vi "NetCDFLabviewDemo.vi"(5 "NetCDF File:":path) -> ()   [LabVIEW 2016]
uses:
  DemoSubVIs/XControls/ArrayTree/ArrayTree.xctl
  DemoSubVIs/XControls/PairTable/PairTable.xctl
panel:
  out "var-lowst-dim name pair":cluster{"name":string, "name":string}[](array[cluster])
  out "DataArr":dbl[][](array[numeric])
  out "Var's Attritutes:":string="No attibutes" caption="valtime's attributes:"
  in  "选项卡控件":enum32{"Global ", "Detail"}(tab)
  out "Global Attritutes":cluster{"c":string, "l":string}[](xcontrol)
  out "Attritutes":cluster{"c":string, "l":string}[](xcontrol)
  out "Variable":T1(xcontrol)
  out "XY图":cluster{dbl[], "value":dbl[]}[](graph) caption="H[0] 's graph"
  in  "ViewPic":bool
  out "Text Variable":string caption="datetime[0](dump text)"
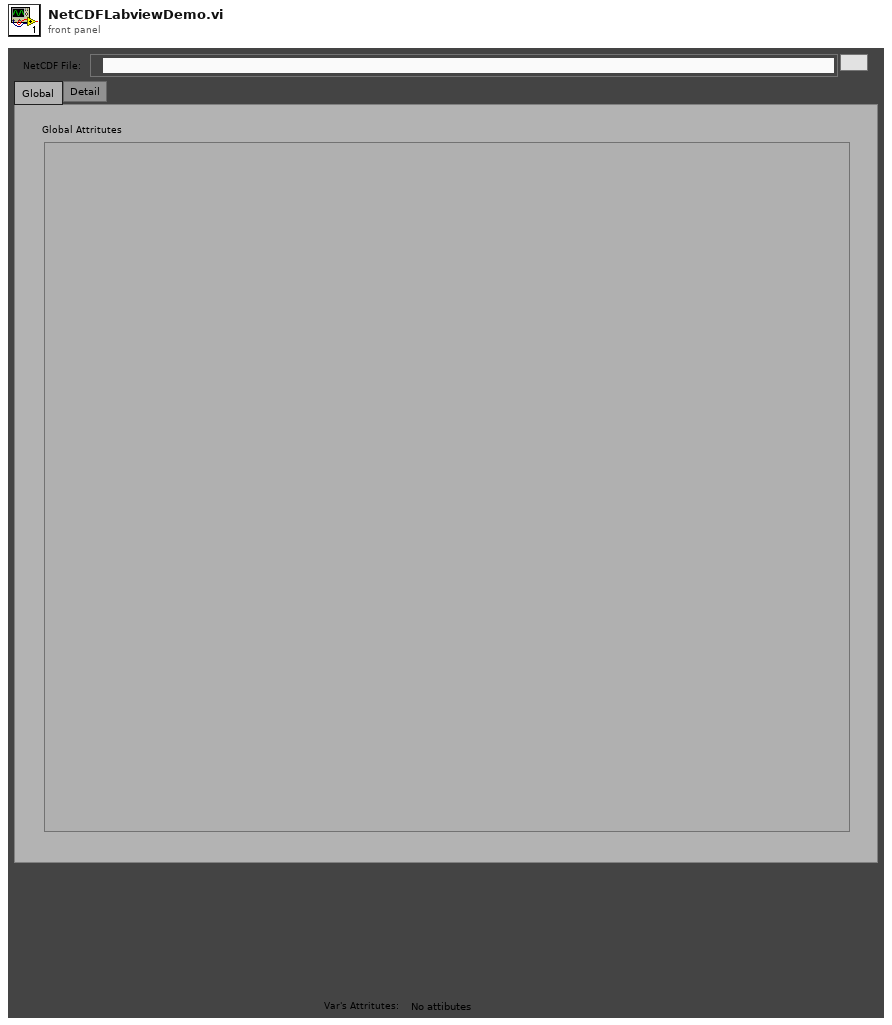
[diagram p1: front panel]
types:
  T1 = cluster{"TopLevelItemName":string, "ChildItemArr":cluster{"ChildDimName":string, "ChildDimSize":u64}[]}[]
  T2 = cluster{"TopLevelItemName":string, "ChildItemArr":cluster{"ChildDimName":string, "ChildDimSize":u64}[]}
  T3 = cluster{"xsz":u64, "shape":u64[], "dsizes":u64[], "name":string, "dimids":u64[], "NC_attrarray":cluster{"xsz":u64, "name":string, "nc_type":u16, "nelems":u64, "xvalue":string}[], "nc_type":enum16{"NC_NAT", "NC_BYTE", "NC_CHAR", "NC_SHORT", "NC_INT", "NC_FLOAT", "NC_DOUBLE"}, "len":u64, "begin":u64}
  T4 = cluster{"xsz":u64, "shape":u64[], "dsizes":u64[], "name":string, "dimids":u64[], "NC_attrarray":cluster{"xsz":u64, "name":string, "nc_type":u16, "nelems":u64, "xvalue":string}[], "nc_type":enum16{"NC_NAT", "NC_BYTE", "NC_CHAR", "NC_SHORT", "NC_INT", "NC_FLOAT", "NC_DOUBLE"}, "len":u64, "begin":u64}[]
  T5 = cluster{"xsz":u64, "name":string, "nc_type":u16, "nelems":u64, "xvalue":string}[]
  T6 = cluster{"numrecs":u64, "dims":cluster{"name":string, "size":u64}[], "attrs":cluster{"xsz":u64, "name":string, "nc_type":u16, "nelems":u64, "xvalue":string}[], "vars":cluster{"xsz":u64, "shape":u64[], "dsizes":u64[], "name":string, "dimids":u64[], "NC_attrarray":cluster{"xsz":u64, "name":string, "nc_type":u16, "nelems":u64, "xvalue":string}[], "nc_type":enum16{"NC_NAT", "NC_BYTE", "NC_CHAR", "NC_SHORT", "NC_INT", "NC_FLOAT", "NC_DOUBLE"}, "len":u64, "begin":u64}[]}
  T7 = enum16{"NC_NAT", "NC_BYTE", "NC_CHAR", "NC_SHORT", "NC_INT", "NC_FLOAT", "NC_DOUBLE"}
  T8 = cluster{"name":string, cluster{"name":string, "数值":u64}[]}[]
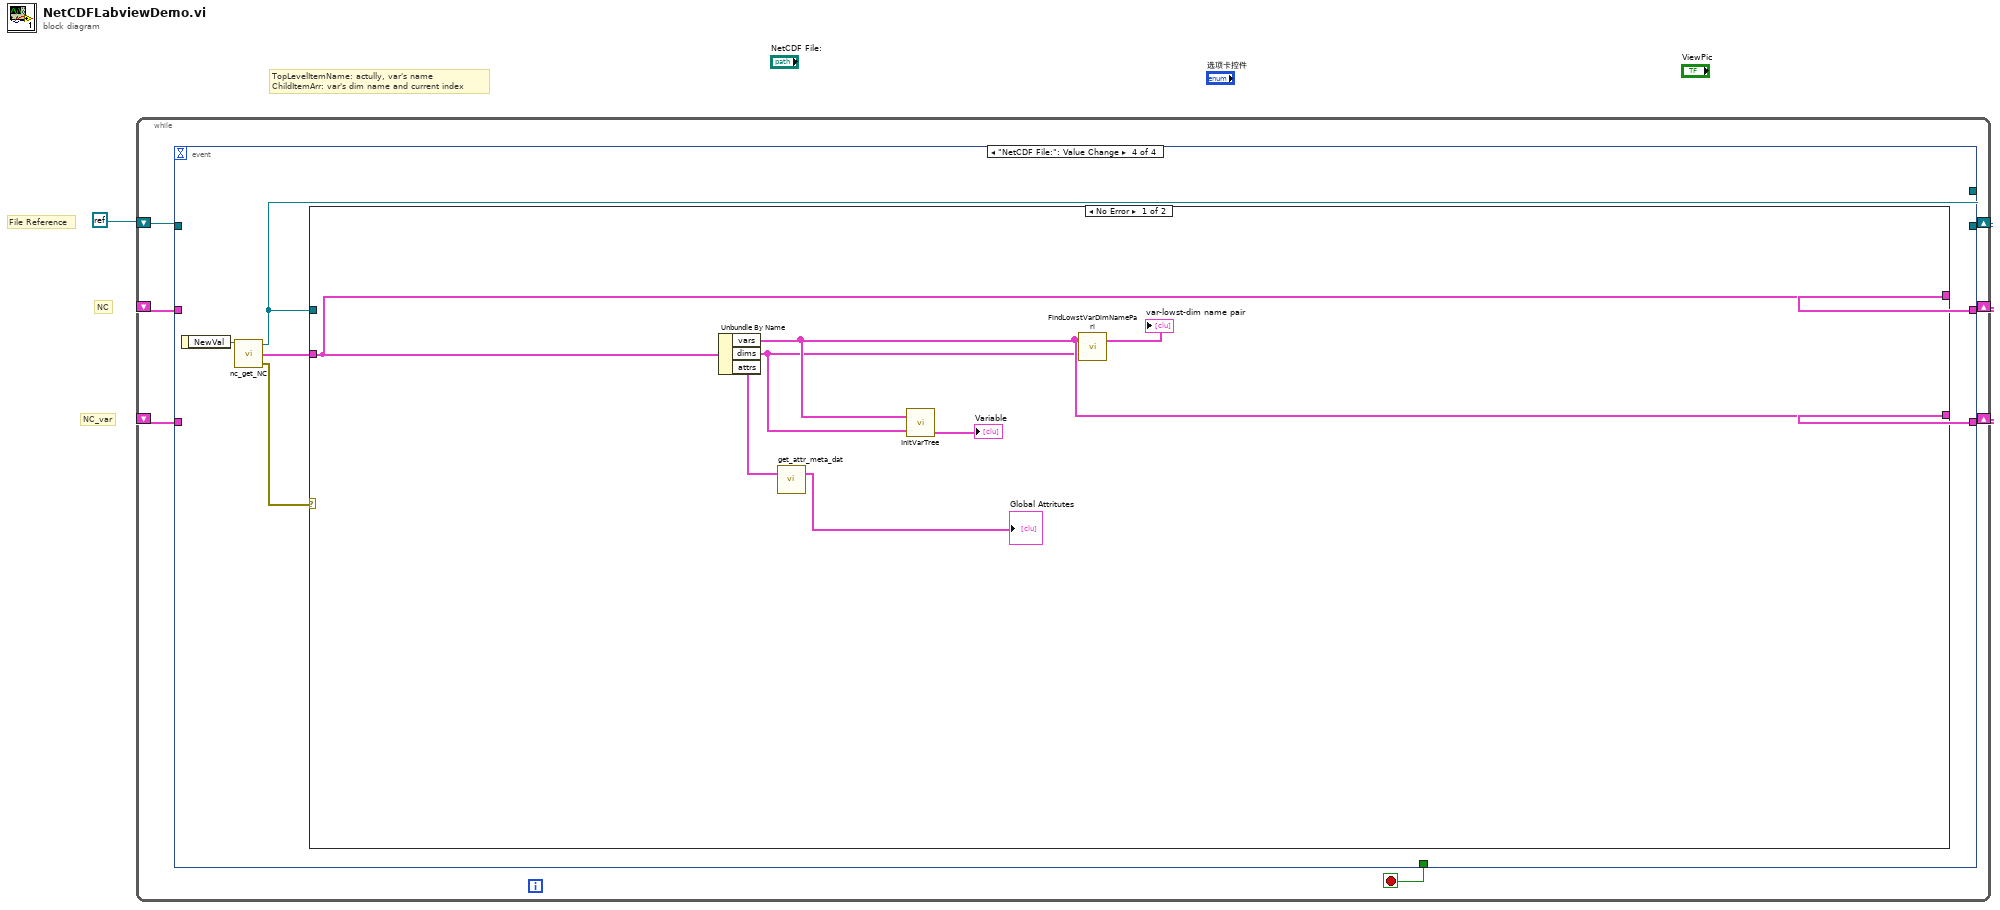
[diagram p0: block diagram]
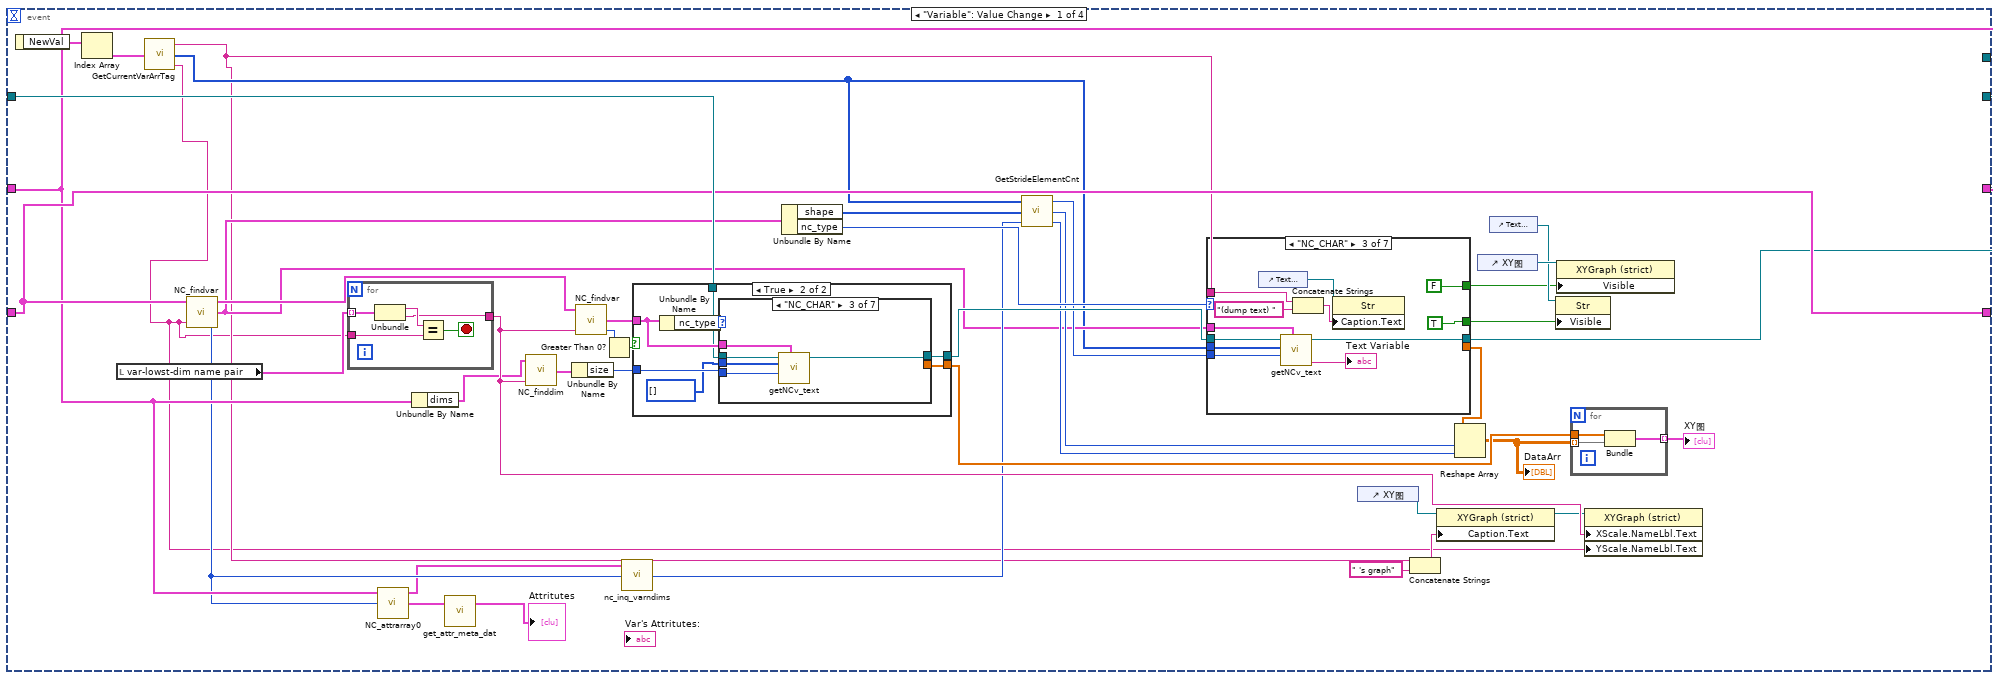
[diagram p2: hidden frame]
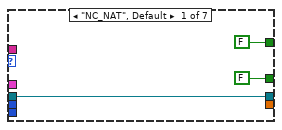
[diagram p3: hidden frame]
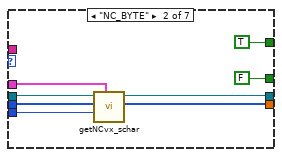
[diagram p4: hidden frame]
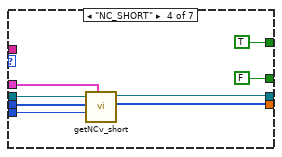
[diagram p5: hidden frame]
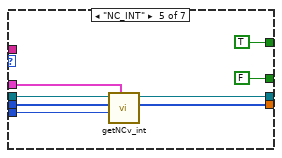
[diagram p6: hidden frame]
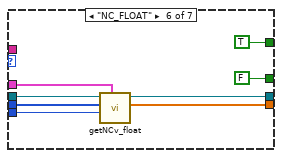
[diagram p7: hidden frame]
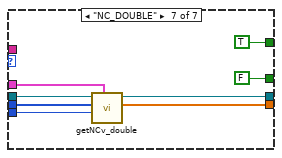
[diagram p8: hidden frame]
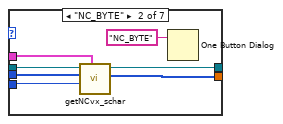
[diagram p11: hidden frame]
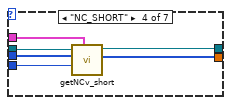
[diagram p12: hidden frame]
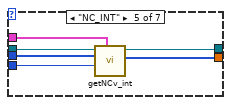
[diagram p13: hidden frame]
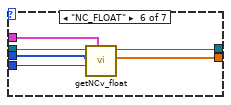
[diagram p14: hidden frame]
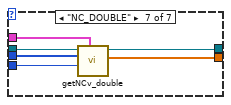
[diagram p15: hidden frame]
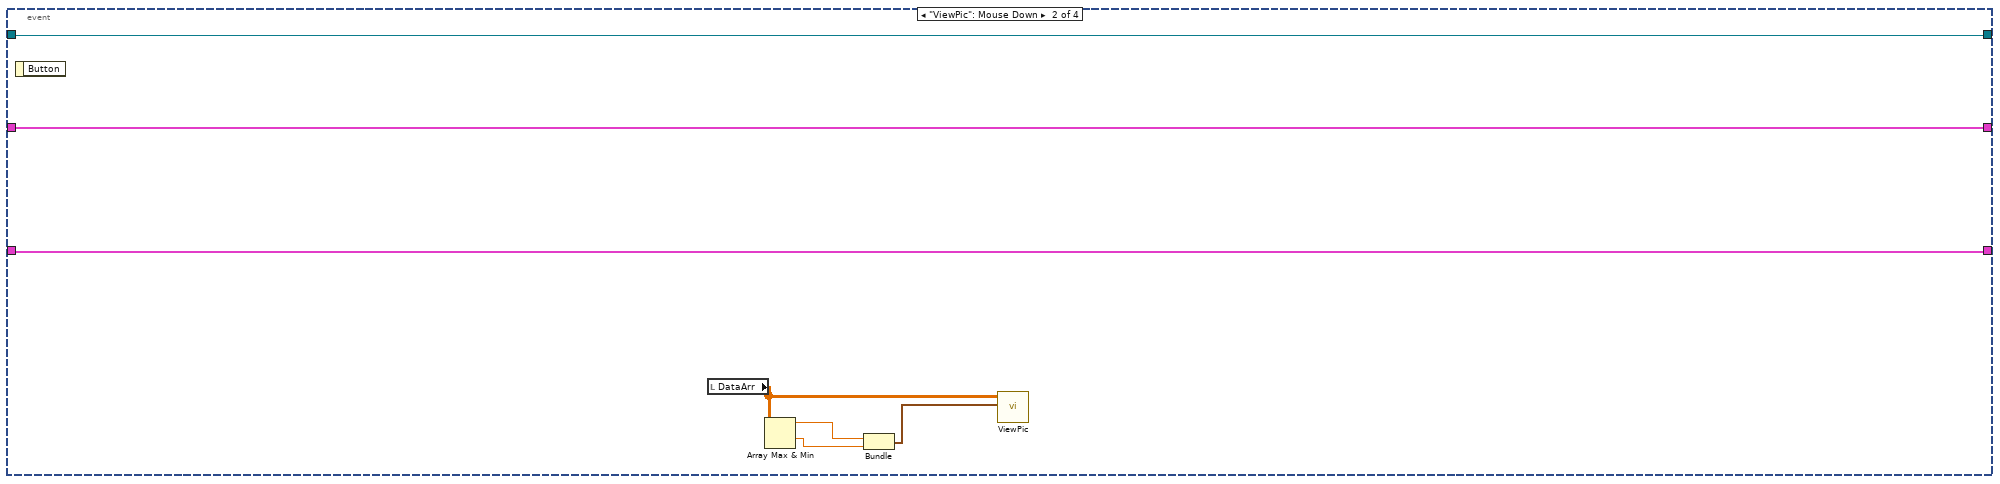
[diagram p16: hidden frame]
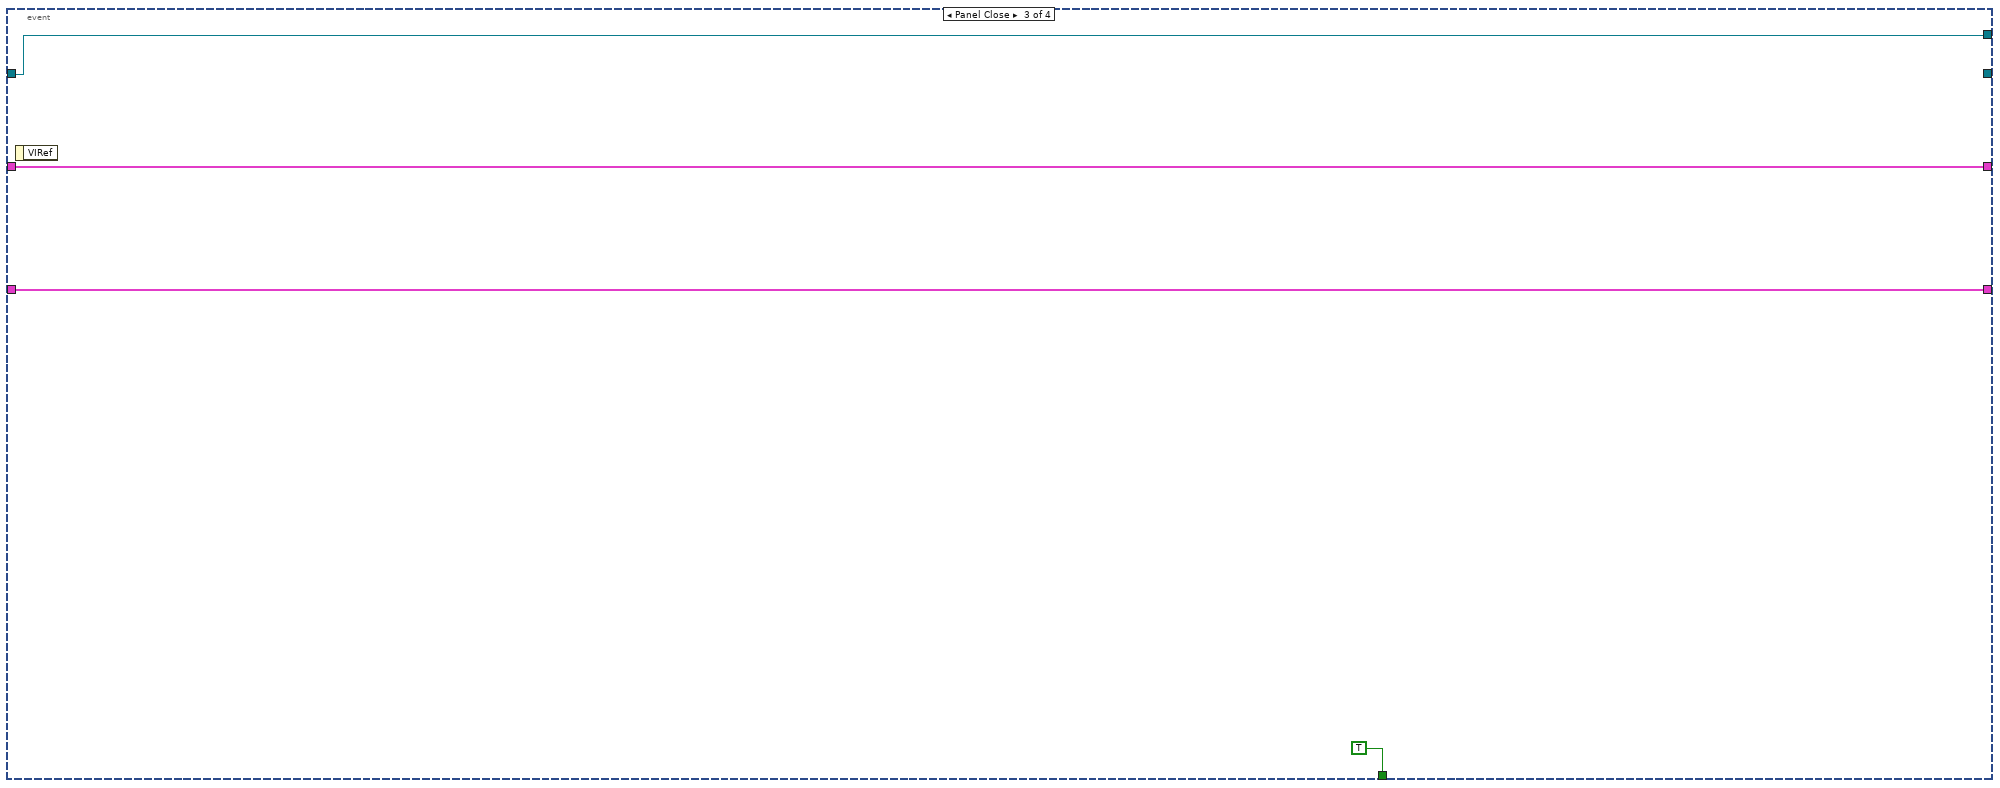
[diagram p17: hidden frame]
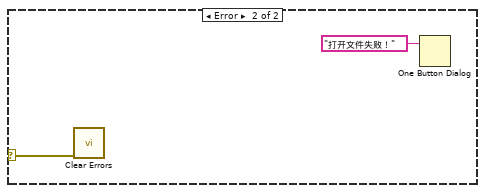
[diagram p18: hidden frame]
diagram:
  # "TopLevelItemName: actully, var's name\nChildItemArr: var's dim name and current index"
  # "File Reference"
  # "NC_var"
  # "NC"
  n1 = while {
    shift-right: [w3] -> _
    shift-left: refnum<k0> refnum -> [w6]
    shift-right: [w5] -> _
    shift-left: _ -> [w7]
    shift-right: [w4] -> _
    shift-left: _ -> [w8]
    stop <- w2 stop-if-true
    n2 = event shown="[3] \"NetCDF File:\": Value Change" {
      selector: _ -> [_ _ _ _]
      dyn-events: _ -> [_ _ _ _]
      timeout: _ -> [_ _ _ _]
      tunnel: w6 -> [w49 w162 w171 _]
      tunnel: w8 -> [w48 w164 w169 _]
      tunnel: w7 -> [w47 w163 w170 _]
      tunnel: [w47 w163 w170 w174] -> w5
      tunnel: [w48 w164 w169 w177] -> w4
      tunnel: [w46 w162 _ w173] -> w3
      tunnel: [_ _ TRUE _] -> w2
      tunnel: [_ _ w171 _] -> _
      event "Variable": Value Change {
        n3 = event-data() -> ("NewVal"=w50:T1)  [unwired: 1 out]
        n4 = Index Array(array=w50) -> (element=w44:T2)  [unwired: 1 in]
        n5 = local read "var-lowst-dim name pair"() -> (w12:cluster{"name":string, "name":string}[])
        n6 = call "GetCurrentVarArrTag.vi"("VarIndexArr"=w44) -> ("CurrentArrayTag"=w11:string, "IndexTagArr"=w14:u64[], "TopLevelItemName"=w10:string)
        n7 = call "NC_findvar.vi"("name"=w10, "NC_vararray"=w48) -> ("varid"=w34:i32, "NC_var"=w15:T3, "NC_vararray  out"=w43:T4)  [unwired: 1 out]
        n8 = for {
          tunnel: w12 -> [w159] mode=indexing
          tunnel: w10 -> [w161]
          tunnel: [w157] -> w41
          stop <- w160 stop-if-true
          n9 = Unbundle(w159) -> ("name"=w158:string, "name"=w157:string)
          n10 = Equal?(x=w158, y=w161) -> (x = y?=w160:bool)
        }
        n11 = call "NC_attrarray0.vi"("varid"=w34, "NC"=w47) -> ("NC_attrarray"=w36:T5, "NC Out"=w32:T6)  [unwired: 1 in, 1 out]
        n12 = Unbundle By Name(w47) -> ("dims"=w35:cluster{"name":string, "size":u64}[])
        n13 = call "get_attr_meta_dat.vi"("NC_attrarray"=w36) -> ("NC_attr_meta_data_arr"=→"Attritutes":cluster{"name":string, "xvalue":string}[])  [unwired: 2 out]
        n14 = call "NC_finddim.vi"("name"=w41, "NC_dimarray"=w35) -> ("NC_dim"=w42:cluster{"name":string, "size":u64})  [unwired: 3 out]
        n15 = Unbundle By Name(w42) -> ("size"=w40:u64)
        n16 = call "NC_findvar.vi"("name"=w41, "NC_vararray"=w43) -> ("varid"=w31:i32, "NC_var"=w39:T3)  [unwired: 2 out]
        n17 = Greater Than 0?(x=w31) -> (x > 0?=w30:bool)
        n18 = call "nc_inq_varndims.vi"("varid"=w34, "NC"=w32) -> ("ndims"=w33:i32)  [unwired: 1 in, 2 out]
        n19 = case shown="True" w30 {
          tunnel: w40 -> [w110 w118]
          tunnel: w39 -> [_ w117]
          tunnel: [w109 w116] -> w38
          tunnel: [w111 w115] -> w37
          tunnel: w49 -> [w111 w114]
          frame False {
            n20 = for {
              N: w110 -> [_]
              tunnel: [w112] -> w109 mode=indexing
              i -> [w112]
            }
          }
          frame True {
            n21 = Unbundle By Name(w117) -> ("nc_type"=w119:T7)
            n22 = case shown="\"NC_CHAR\"" w119 {
              tunnel: [_ w124 _ w137 w142 w147 w153] -> w116
              tunnel: w114 -> [w120 w126 w131 w138 w144 w150 w156]
              tunnel: w118 -> [_ w122 w130 w136 w143 w149 w155]
              tunnel: w117 -> [_ w125 w132 w135 w141 w148 w154]
              tunnel: [w120 w123 w129 w134 w140 w146 w152] -> w115
              tunnel: u64[] [] ("start") -> [_ w121 w128 w133 w139 w145 w151]
              frame "NC_NAT", Default {
              }
              frame "NC_BYTE" {
                n23 = call "getNCvx_schar.vi"("NC_var"=w125, "nelems"=w122, "start"=w121, "refnum"=w126) -> ("value"=w124:i8[], "refnum out"=w123:refnum<file>)  [unwired: 1 in, 2 out]
                n24 = One Button Dialog(message="NC_BYTE" ("消息")) -> ()  [unwired: 2 out]
              }
              frame "NC_CHAR" {
                n25 = call "getNCv_text.vi"("NC_var"=w132, "nelems"=w130, "start"=w128, "refnum"=w131) -> ("refnum out"=w129:refnum<file>)  [unwired: 1 in, 3 out]
              }
              frame "NC_SHORT" {
                n26 = call "getNCv_short.vi"("NC_var"=w135, "nelems"=w136, "start"=w133, "refnum"=w138) -> ("value"=w137:i16[], "refnum out"=w134:refnum<file>)  [unwired: 1 in, 2 out]
              }
              frame "NC_INT" {
                n27 = call "getNCv_int.vi"("NC_var"=w141, "nelems"=w143, "start"=w139, "refnum"=w144) -> ("value"=w142:i32[], "refnum out"=w140:refnum<file>)  [unwired: 1 in, 2 out]
              }
              frame "NC_FLOAT" {
                n28 = call "getNCv_float.vi"("NC_var"=w148, "nelems"=w149, "start"=w145, "refnum"=w150) -> ("value"=w147:sgl[], "refnum out"=w146:refnum<file>)  [unwired: 1 in, 2 out]
              }
              frame "NC_DOUBLE" {
                n29 = call "getNCv_double.vi"("NC_var"=w154, "nelems"=w155, "start"=w151, "refnum"=w156) -> ("value"=w153:dbl[], "refnum out"=w152:refnum<file>)  [unwired: 1 in, 2 out]
              }
            }
          }
        }
        n30 = Unbundle By Name(w15) -> ("shape"=w13:u64[], "nc_type"=w45:T7)
        n31 = call "GetStrideElementCnt.vi"("ndims"=w33, "shape"=w13, "CurrentIndex"=w14) -> ("shape[i-1]"=w29:u64, "shape[i-2]"=w28:u64, "strideElementCnt"=w16:u64)
        n32 = case shown="\"NC_CHAR\"" w45 {
          tunnel: [_ w60 _ w83 w89 w96 w104] -> w27
          tunnel: w37 -> [w56 w64 w74 w84 w92 w100 w108]
          tunnel: w16 -> [_ w61 w72 w82 w90 w98 w106]
          tunnel: w11 -> [_ _ w68 _ _ _ _]
          tunnel: w14 -> [_ w62 w73 w80 w91 w99 w107]
          tunnel: w15 -> [_ w63 w75 w81 w88 w97 w105]
          tunnel: [w56 w59 w70 w79 w87 w95 w103] -> w46
          tunnel: [FALSE ("可见") TRUE ("可见") FALSE ("可见") TRUE ("可见") TRUE ("可见") TRUE ("可见") TRUE ("可见")] -> w20
          tunnel: [FALSE ("可见") FALSE ("可见") TRUE ("可见") FALSE ("可见") FALSE ("可见") FALSE ("可见") FALSE ("可见")] -> w19
          frame "NC_NAT", Default {
          }
          frame "NC_BYTE" {
            n33 = call "getNCvx_schar.vi"("NC_var"=w63, "nelems"=w61, "start"=w62, "refnum"=w64) -> ("value"=w60:i8[], "refnum out"=w59:refnum<file>)  [unwired: 1 in, 2 out]
          }
          frame "NC_CHAR" {
            n34 = control-ref of="Text Variable"() -> (w76:refnum<vi>)
            n35 = call "getNCv_text.vi"("NC_var"=w75, "nelems"=w72, "start"=w73, "refnum"=w74) -> ("value"=→"Text Variable":string, "refnum out"=w70:refnum<file>)  [unwired: 1 in, 2 out]
            n36 = Concatenate Strings(w68, "(dump text) " ("字符串")) -> (w67:string)
            n37 = property class="Str"(reference=w76, "Caption.Text"=w67) -> ()  [unwired: 1 in, 2 out]
          }
          frame "NC_SHORT" {
            n38 = call "getNCv_short.vi"("NC_var"=w81, "nelems"=w82, "start"=w80, "refnum"=w84) -> ("value"=w83:i16[], "refnum out"=w79:refnum<file>)  [unwired: 1 in, 2 out]
          }
          frame "NC_INT" {
            n39 = call "getNCv_int.vi"("NC_var"=w88, "nelems"=w90, "start"=w91, "refnum"=w92) -> ("value"=w89:i32[], "refnum out"=w87:refnum<file>)  [unwired: 1 in, 2 out]
          }
          frame "NC_FLOAT" {
            n40 = call "getNCv_float.vi"("NC_var"=w97, "nelems"=w98, "start"=w99, "refnum"=w100) -> ("value"=w96:sgl[], "refnum out"=w95:refnum<file>)  [unwired: 1 in, 2 out]
          }
          frame "NC_DOUBLE" {
            n41 = call "getNCv_double.vi"("NC_var"=w105, "nelems"=w106, "start"=w107, "refnum"=w108) -> ("value"=w104:dbl[], "refnum out"=w103:refnum<file>)  [unwired: 1 in, 2 out]
          }
        }
        n42 = control-ref of="XY图"() -> (w26:refnum<vi>)
        n43 = Concatenate Strings(w11, " 's graph" ("字符串")) -> (w17:string)
        n44 = property class="XYGraph (strict)"(reference=w26, "Caption.Text"=w17) -> (reference out=w23:refnum<vi>)  [unwired: 1 in, 1 out]
        n45 = Reshape Array(w27, w28, w29) -> (w25:dbl[][])
        "DataArr" <- w25
        n46 = control-ref of="XY图"() -> (w22:refnum<vi>)
        n47 = control-ref of="Text Variable"() -> (w21:refnum<vi>)
        n48 = property class="Str"(reference=w21, "Visible"=w19) -> ()  [unwired: 1 in, 2 out]
        n49 = property class="XYGraph (strict)"(reference=w22, "Visible"=w20) -> ()  [unwired: 1 in, 2 out]
        n50 = for {
          tunnel: w25 -> [w52] mode=indexing
          tunnel: [w53] -> w24 mode=indexing
          tunnel: w38 -> [w51]
          n51 = Bundle("value"=w51, "value"=w52) -> (w53:cluster{"value":dbl[], "value":dbl[]})  [unwired: 1 out]
        }
        "XY图" <- w24
        n52 = property class="XYGraph (strict)"(reference=w23, "XScale.NameLbl.Text"=w41, "YScale.NameLbl.Text"=w10) -> ()  [unwired: 1 in, 2 out]
      }
      event "ViewPic": Mouse Down {
        n53 = event-data() -> ()  [unwired: 2 out]
        n54 = local read "DataArr"() -> (w168:dbl[][])
        n55 = Array Max & Min(array=w168) -> (max value=w167:dbl, min value=w166:dbl)  [unwired: 2 out]
        n56 = Bundle(w167, w166) -> (w165:cluster{dbl, dbl})  [unwired: 1 out]
        n57 = call "ViewPic.vi"("VarRange"=w165, "Data"=w168) -> ()  [unwired: 1 in, 9 out]
      }
      event Panel Close {
        n58 = event-data() -> ()  [unwired: 2 out]
      }
      event "NetCDF File:": Value Change {
        n59 = event-data() -> ("NewVal"=w178:path)  [unwired: 1 out]
        n60 = call "nc_get_NC.vi"("FilePath"=w178) -> ("ErrorOut"=w176:errorcluster, "NC"=w175:T6, "refnum out"=w173:refnum<file>)  [unwired: 1 in, 1 out]
        n61 = case shown="No Error" w176 {
          selector: w176 -> [_ w186]
          tunnel: [w181 _] -> w177
          tunnel: w175 -> [w182 _]
          tunnel: [w182 _] -> w174
          tunnel: w173 -> [_ _]
          frame No Error {
            n62 = Unbundle By Name(w182) -> ("vars"=w181:T4, "dims"=w180:cluster{"name":string, "size":u64}[], "attrs"=w185:T5)
            n63 = call "get_attr_meta_dat.vi"("NC_attrarray"=w185) -> ("NC_attr_meta_data_arr"=→"Global Attritutes":cluster{"name":string, "xvalue":string}[])  [unwired: 1 in, 1 out]
            n64 = call "InitVarTree.vi"("dims"=w180, "vars"=w181) -> ("var tree"=→"Variable":T8)
            n65 = call "FindLowstVarDimNamePari.vi"("dims"=w180, "vars"=w181) -> ("var-lowst-dim name pair"=→"var-lowst-dim name pair":cluster{"name":string, "name":string}[])
          }
          frame Error {
            n66 = call <vilib>:"Clear Errors.vi"("error in (no error)"=w186) -> ()  [unwired: 1 in, 6 out]
            n67 = One Button Dialog(message="打开文件失败！" ("消息")) -> ()  [unwired: 2 out]
          }
        }
      }
    }
  }
